vi "generate.vi"(8 "error in (no error)":errorcluster, 10 "measurement_conditioning":refnum<class "MeasurementDatalvclass.lvclass">, 11 "Measurement in":refnum<class "Measurement.lvclass">) -> (0 "error out":errorcluster, 3 "Measurement out":refnum<class "Measurement.lvclass">)   [LabVIEW 2017, in "Measurement.lvclass"]
doc: "Generate data needed for the measurement"
uses:
  Measurement.lvclass
  measurement_data/MeasurementDatalvclass.lvclass
  Measurement.lvclass/Measurement.ctl
  hardware/Hardware.lvclass
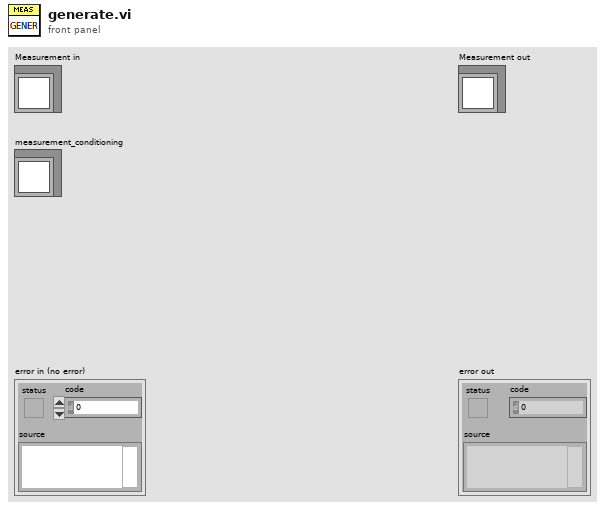
[diagram p1: front panel]
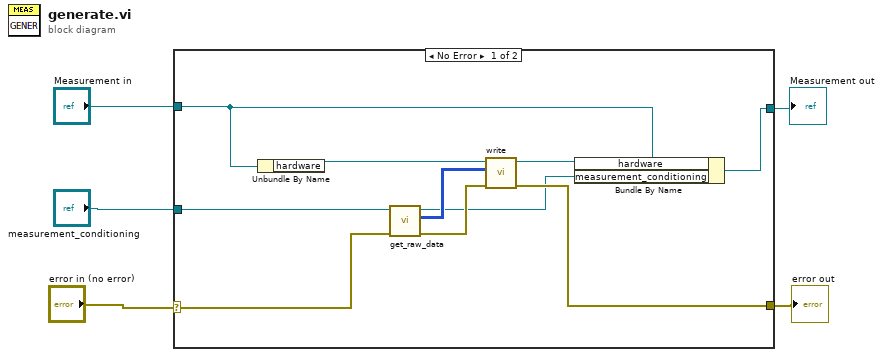
[diagram p0: block diagram]
diagram:
  n1 = case shown="No Error" "error in (no error)" {
    selector: "error in (no error)" -> [w9 w17]
    tunnel: [w8 w17] -> w4
    tunnel: [w10 w16] -> w2
    tunnel: "Measurement in" -> [w11 w16]
    tunnel: "measurement_conditioning" -> [w7 _]
    frame No Error {
      n2 = Unbundle By Name(w11) -> ("hardware"=w15:refnum<class "Hardware.lvclass">)
      n3 = call-dynamic "get_raw_data.vi"("error in (no error)"=w9, "MeasurementResult in"=w7) -> ("error out"=w13:errorcluster, "raw_data"=w14:u16[][], "MeasurementResult out"=w6:refnum<class "MeasurementDatalvclass.lvclass">)  [unwired: 7 in]
      n4 = call-dynamic "write.vi"("error in (no error)"=w13, "inputs"=w14, "Hardware in"=w15) -> ("error out"=w8:errorcluster, "Hardware out"=w12:refnum<class "Hardware.lvclass">)  [unwired: 7 in]
      n5 = Bundle By Name(cluster=w11, "hardware"=w12, "measurement_conditioning"=w6) -> (w10:refnum<class "Measurement.lvclass">)
    }
    frame Error {
    }
  }
  "error out" <- w4
  "Measurement out" <- w2
